vi "Write angle.vi"(8 "error in (no error)":errorcluster, 10 "angle":dbl[unit], 11 "Position in":refnum<class "Position.lvclass">) -> (0 "error out":errorcluster, 3 "Position out":refnum<class "Position.lvclass">)   [LabVIEW 2016, in "UnitsAndXML.lvlib" / "Position.lvclass"]
uses:
  <userlib>/Common/UnitsAndXML/SupportFiles/Position/Position.lvclass
  <userlib>/Common/UnitsAndXML/SupportFiles/Position/Position.lvclass/Position.ctl
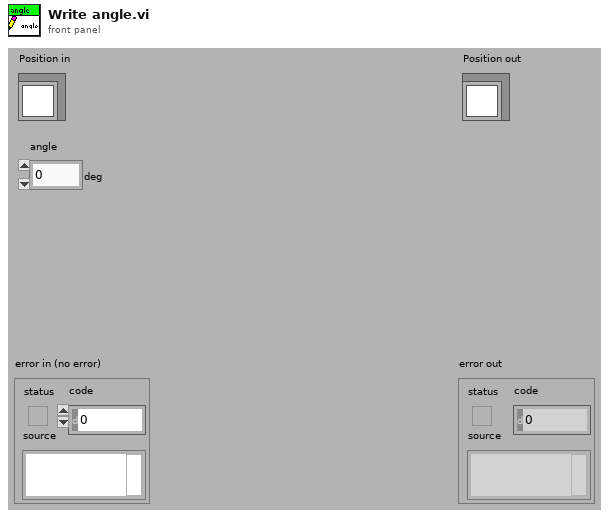
[diagram p1: front panel]
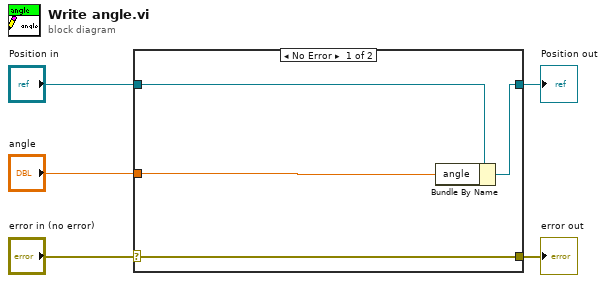
[diagram p0: block diagram]
diagram:
  n1 = case shown="No Error" "error in (no error)" {
    selector: "error in (no error)" -> [w9 w10]
    tunnel: [w9 w10] -> w4
    tunnel: [w7 w11] -> w2
    tunnel: "Position in" -> [w8 w11]
    tunnel: "angle" -> [w6 _]
    frame No Error {
      n2 = Bundle By Name(cluster=w8, "angle"=w6) -> (w7:refnum<class "Position.lvclass">)
    }
    frame Error {
    }
  }
  "error out" <- w4
  "Position out" <- w2
